vi "Write port.vi"(8 "error in (no error)":errorcluster, 10 "port":u16, 11 "URI in":refnum<class "URI.lvclass">) -> (0 "error out":errorcluster, 3 "URI out":refnum<class "URI.lvclass">)   [LabVIEW 2013, in "openURI.lvlib" / "URI.lvclass"]
uses:
  URI.lvclass
  URI.lvclass/URI.ctl
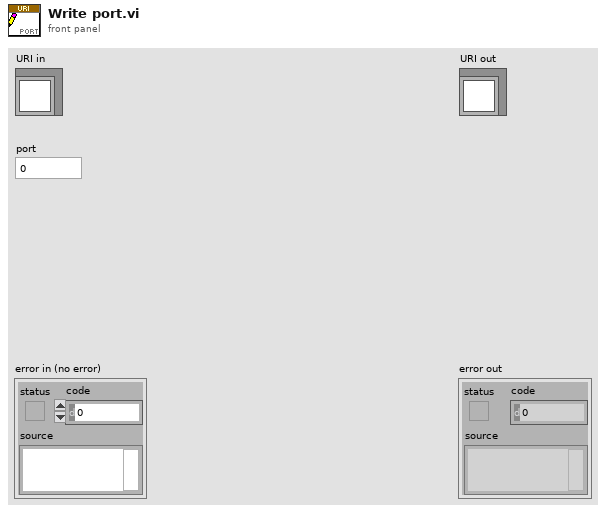
[diagram p1: front panel]
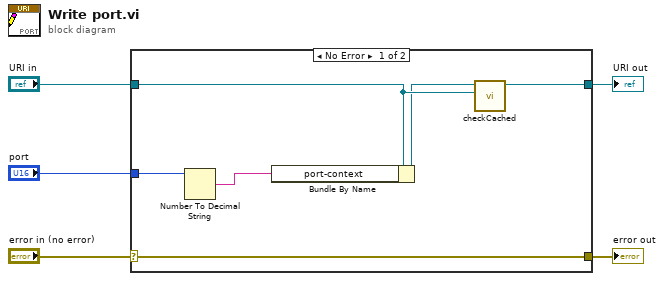
[diagram p0: block diagram]
diagram:
  n1 = case shown="No Error" "error in (no error)" {
    selector: "error in (no error)" -> [w11 w12]
    tunnel: [w11 w12] -> w4
    tunnel: [w8 w13] -> w2
    tunnel: "URI in" -> [w10 w13]
    tunnel: "port" -> [w7 _]
    frame No Error {
      n2 = Number To Decimal String(number=w7) -> (decimal integer string=w6:string)  [unwired: 1 in]
      n3 = Bundle By Name(cluster=w10, "port-context"=w6) -> (w9:refnum<class "URI.lvclass">)
      n4 = call "checkCached.vi"("Old"=w10, "New URI"=w9) -> ("URI"=w8:refnum<class "URI.lvclass">)  [unwired: 9 in]
    }
    frame Error {
    }
  }
  "error out" <- w4
  "URI out" <- w2
